vi "Get SMO HELP.vi"(8 "error in (no error)":errorcluster, 10 "Command":string, 11 "Instrument in":refnum<class "Instrument.lvclass">) -> (0 "error out":errorcluster, 2 "help cluster":T1, 3 "Instrument out":refnum<class "Instrument.lvclass">)   [LabVIEW 2019, in "Instrument.lvclass"]
uses:
  Instrument.lvclass
  Help/typedefs/Help--cluster.ctl
  Typedefs/Instrument.Commands--Enum.ctl
  Typedefs/Instrument.IDN--cluster.ctl
  Help/Help.lvclass
  subsystems/JSON-Schema/JSON-Schema/JSON-Schema.lvlib
  <vilib>/JKI/JKI SMO/SMO/SMO.lvclass
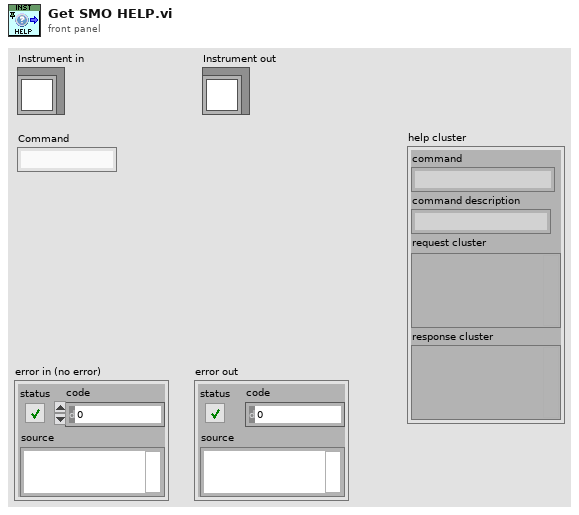
[diagram p1: front panel]
types:
  T1 = typedef "Help.lvclass/Help--cluster.ctl" = cluster{"command":string, "command description":string, "request cluster":variant, "response cluster":variant}
  T2 = typedef "Instrument.lvclass/Instrument.Commands--Enum.ctl" = enum16{"ACK", "HELP", "IDN", "getAll", "getAllData"}
  T3 = typedef "Instrument.lvclass/Instrument.IDN--cluster.ctl" = cluster{"vendor":string, "model":string, "serial":string, "firmware":string}
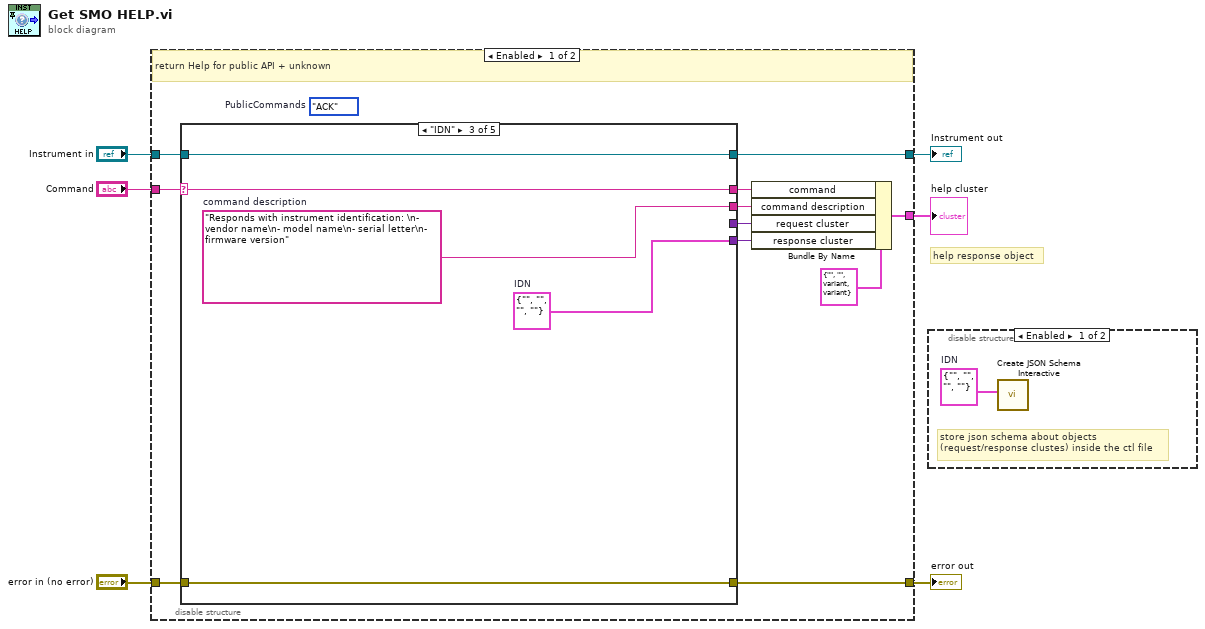
[diagram p0: block diagram]
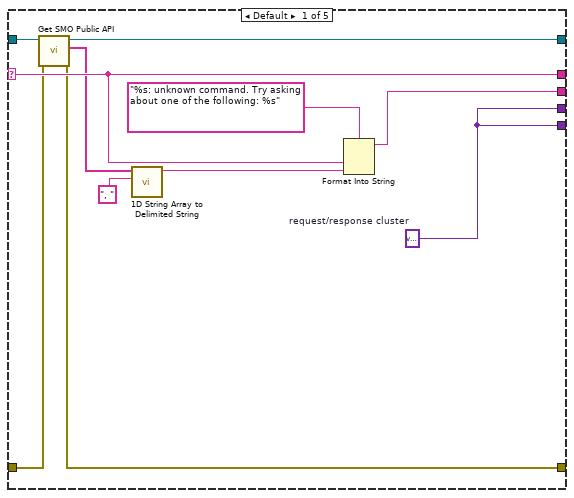
[diagram p3: hidden frame]
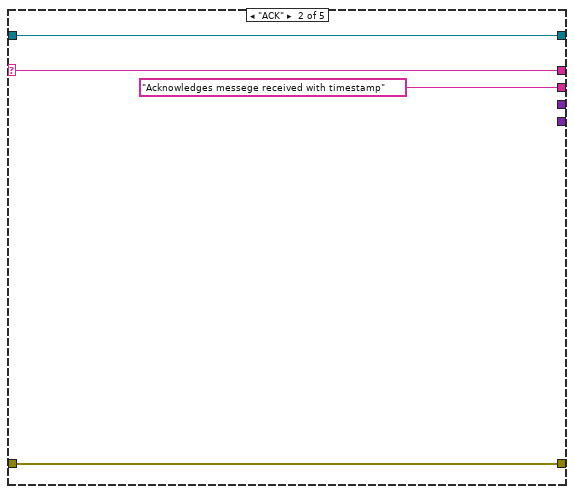
[diagram p4: hidden frame]
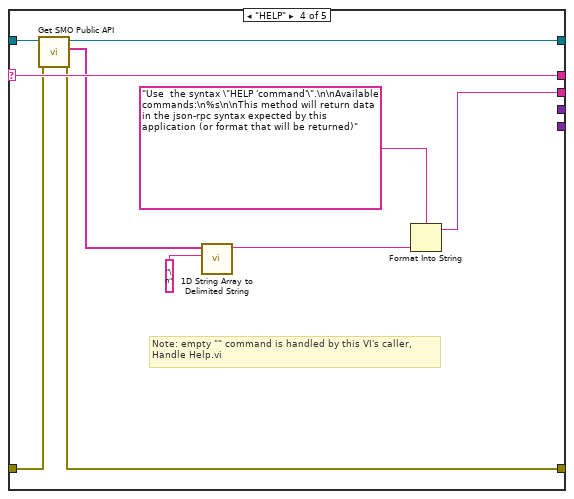
[diagram p5: hidden frame]
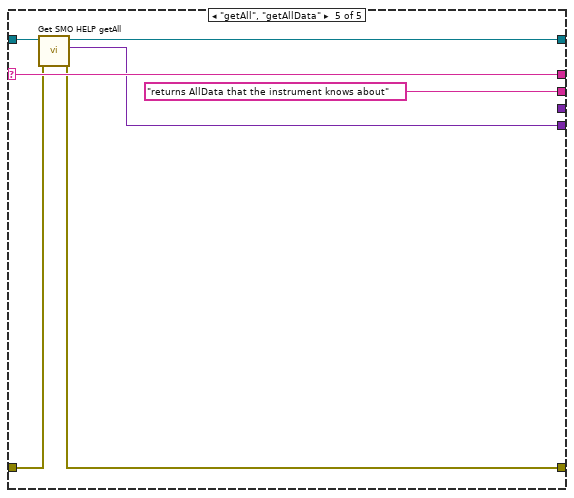
[diagram p6: hidden frame]
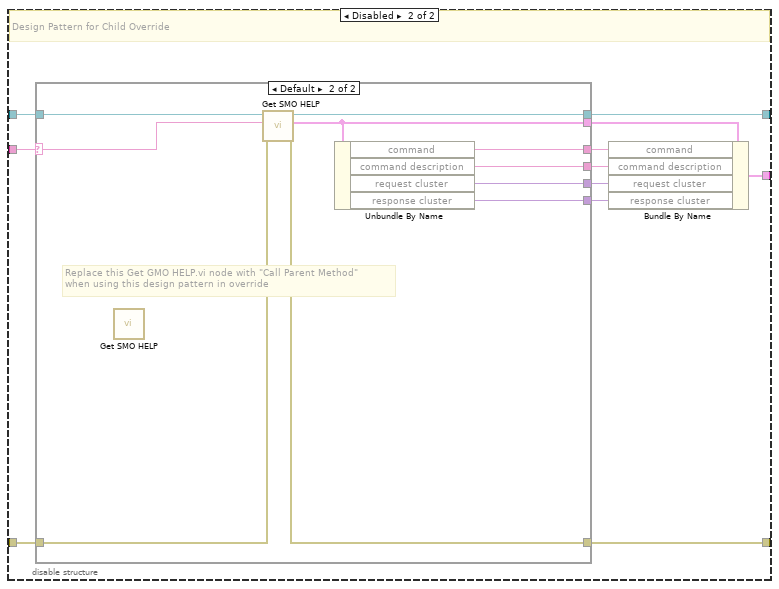
[diagram p7: hidden frame]
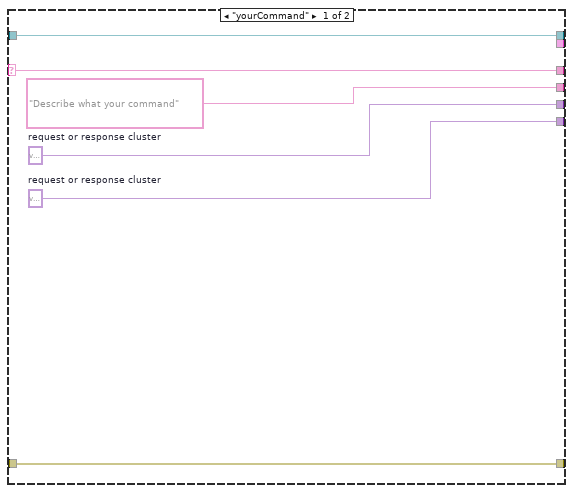
[diagram p8: hidden frame]
diagram:
  # "help response object"
  n1 = disable-structure shown="Enabled" {
    disable-tunnel: [w17 w56] -> w6
    disable-tunnel: "Instrument in" -> [w16 w57]
    disable-tunnel: "error in (no error)" -> [w15 w63]
    disable-tunnel: [w11 w65] -> w3
    disable-tunnel: [w8 w64] -> w2
    disable-tunnel: "Command" -> [w7 w62]
    frame Enabled {
      (unwired) Instrument.Commands--Enum."ACK"  # PublicCommands
      # "return Help for public API + unknown"
      n2 = case shown="\"IDN\"" w7 {
        selector: w7 -> [w24 w30 w36 w44 w53]
        tunnel: w15 -> [w21 w32 w34 w40 w52]
        tunnel: [w22 w32 w34 w41 w51] -> w11
        tunnel: [w26 "Acknowledges messege received with timestamp" w37 w43 "returns AllData that the instrument knows about"] -> w13
        tunnel: [w19 _ _ _ _] -> w12
        tunnel: [w19 _ w33 _ w48] -> w10
        tunnel: [w24 w30 w36 w44 w53] -> w14
        tunnel: w16 -> [w23 w29 w35 w42 w49]
        tunnel: [w20 w29 w35 w39 w50] -> w17
        frame Default {
          w19 = variant  # request/response cluster
          n3 = call-dynamic "Get SMO Public API.vi"("error in (no error)"=w21, "Instrument in"=w23) -> ("error out"=w22:errorcluster, "commands"=w18:string[], "Instrument out"=w20:refnum<class "Instrument.lvclass">)  [unwired: 7 in]
          n4 = call <vilib>:"1D String Array to Delimited String.vi"("delimiter"=", ", "string array"=w18) -> ("delimited string"=w27:string)  [unwired: 9 in]
          n5 = Format Into String(format string="%s: unknown command. Try asking about one of the following: %s", w24, w27) -> (resulting string=w26:string)  [unwired: 2 in, 1 out]
        }
        frame "ACK" {
        }
        frame "IDN" {
          w33 = T3 {"vendor"="", "model"="", "serial"="", "firmware"=""}  # IDN
          w37 = "Responds with instrument identification: \n- vendor name\n- model name\n- serial letter\n- firmware version"  # command description
        }
        frame "HELP" {
          # "Note: empty \"\" command is handled by this VI's caller,\nHandle Help.vi"
          n6 = call-dynamic "Get SMO Public API.vi"("error in (no error)"=w40, "Instrument in"=w42) -> ("error out"=w41:errorcluster, "commands"=w38:string[], "Instrument out"=w39:refnum<class "Instrument.lvclass">)  [unwired: 7 in]
          n7 = call <vilib>:"1D String Array to Delimited String.vi"("delimiter"="\n", "string array"=w38) -> ("delimited string"=w47:string)  [unwired: 9 in]
          n8 = Format Into String(format string="Use  the syntax \"HELP 'command'\".\n\nAvailable commands:\n%s\n\nThis method will return data in the json-rpc syntax expected by this application (or format that will be returned)", w47) -> (resulting string=w43:string)  [unwired: 2 in, 1 out]
        }
        frame "getAll", "getAllData" {
          n9 = call-dynamic "Get SMO HELP getAll.vi"("error in (no error)"=w52, "Instrument in"=w49) -> ("error out"=w51:errorcluster, "response cluster"=w48:variant, "Instrument out"=w50:refnum<class "Instrument.lvclass">)  [unwired: 7 in]
        }
      }
      n10 = Bundle By Name(cluster=T1 {"command"="", "command description"="", "request cluster"=variant, "response cluster"=variant} ("Help"), "command"=w14, "command description"=w13, "request cluster"=w12, "response cluster"=w10) -> (w8:T1)
    }
    frame Disabled {
      # "Design Pattern for Child Override"
      n11 = case shown="Default" w62 {
        selector: w62 -> [w71 w80]
        tunnel: [w71 w75] -> w61
        tunnel: w63 -> [w70 w73]
        tunnel: [w70 w72] -> w65
        tunnel: ["Describe what your command" w76] -> w60
        tunnel: [w68 w77] -> w59
        tunnel: [w67 w78] -> w58
        tunnel: w57 -> [w66 w81]
        tunnel: [w66 w79] -> w56
        tunnel: [_ w74] -> w55
        frame "yourCommand" {
          w68 = variant  # request or response cluster
          w67 = variant  # request or response cluster
        }
        frame Default {
          # "Replace this Get GMO HELP.vi node with \"Call Parent Method\"\nwhen using this design pattern in override"
          n12 = call-parent "Get SMO HELP.vi"() -> ()  [unwired: 1 in]
          n13 = call-dynamic "Get SMO HELP.vi"("error in (no error)"=w73, "Command"=w80, "Instrument in"=w81) -> ("error out"=w72:errorcluster, "help cluster"=w74:T1, "Instrument out"=w79:refnum<class "Instrument.lvclass">)  [unwired: 6 in]
          n14 = Unbundle By Name(w74) -> ("command"=w75:string, "command description"=w76:string, "request cluster"=w77:variant, "response cluster"=w78:variant)
        }
      }
      n15 = Bundle By Name(cluster=w55, "command"=w61, "command description"=w60, "request cluster"=w59, "response cluster"=w58) -> (w64:T1)
    }
  }
  "Instrument out" <- w6
  "help cluster" <- w2
  "error out" <- w3
  n16 = disable-structure shown="Enabled" {
    frame Enabled {
      w82 = T3 {"vendor"="", "model"="", "serial"="", "firmware"=""}  # IDN
      # "store json schema about objects\n(request/response clustes) inside the ctl file"
      n17 = call "Create JSON Schema Interactive.vi"("LV Object"=w82) -> ()  [unwired: 9 in, 2 out]
    }
    frame Disabled {
    }
  }
